vi "settings ui.vi"(10 "ActorConfiguration":T5={"GlobalConfiguration"={"DeviceFamily"="", "WriteData"=FALSE, "BufferSize_samples"=-1, "SyncDevice"=FALSE, "ExecuteInterruptRoutine"=FALSE, "InterruptRoutineTimeout_ms"=-1}, "DeviceConfiguration"={"DeviceSpecificName"="MIPI_Camera", "HardwareReference"="PXIe-Slot2", "UsedResources"=[{"ResourceLocation"="FrontFacing", "ResourceData"=variant(string "Use this Variant to store your specific resource data.\nThis will be read from and written to with the JSON parsing API.\nIn the child implementation you can use the acessors provided to convert from the specific cluster to your own device's implementation")}]}}, 11 "Template":refnum<class "Template.lvclass">) -> (0 "error out":errorcluster, 2 "ActorConfiguration":T5={"GlobalConfiguration"={"DeviceFamily"="", "WriteData"=FALSE, "BufferSize_samples"=-1, "SyncDevice"=FALSE, "ExecuteInterruptRoutine"=FALSE, "InterruptRoutineTimeout_ms"=-1}, "DeviceConfiguration"={"DeviceSpecificName"="MIPI_Camera", "HardwareReference"="PXIe-Slot2", "UsedResources"=[{"ResourceLocation"="FrontFacing", "ResourceData"=variant(string "Use this Variant to store your specific resource data.\nThis will be read from and written to with the JSON parsing API.\nIn the child implementation you can use the acessors provided to convert from the specific cluster to your own device's implementation")}]}})   [LabVIEW 2020, in "Template.lvlib" / "Template.lvclass"]
doc: "Overrides the UI implementation of the settings definition.\nReturns the new configuration for the update settings.vi method"
uses:
  Template.lvclass
  typedefs/actor configuration.ctl
  typedefs/shared actor configuration.ctl
  typedefs/resource config/device configuration cluster.ctl
  typedefs/resource config/single resource cluster.ctl
  f39a1763-17d9-4e4e-a317-0c97e162ffb7.vi
  f86444c9-f386-4375-ae10-303c8fbaebf9.vi
  <vilib>/JDP Science/JSONtext/JSON text to Variant.vi
  <vilib>/JDP Science/JSONtext/Variant to JSON Text.vi
  <vilib>/JDP Science/JSONtext/LVClass Serializer/JSONtext LVClass Serializer.lvclass
panel:
  in  "Sample Resource Data":T1(array[cluster])
  out "Valid JSON?":bool
  in  "JSON Text":string
  in  "DeviceConfiguration":T2={"DeviceSpecificName"="MIPI_Camera", "HardwareReference"="PXIe-Slot2", "UsedResources"=[{"ResourceLocation"="FrontFacing", "ResourceData"=variant(string "Use this Variant to store your specific resource data.\nThis will be read from and written to with the JSON parsing API.\nIn the child implementation you can use the acessors provided to convert from the specific cluster to your own device's implementation")}]}
  in  "GlobalConfiguration":T4={"DeviceFamily"="", "WriteData"=FALSE, "BufferSize_samples"=-1, "SyncDevice"=FALSE, "ExecuteInterruptRoutine"=FALSE, "InterruptRoutineTimeout_ms"=-1}
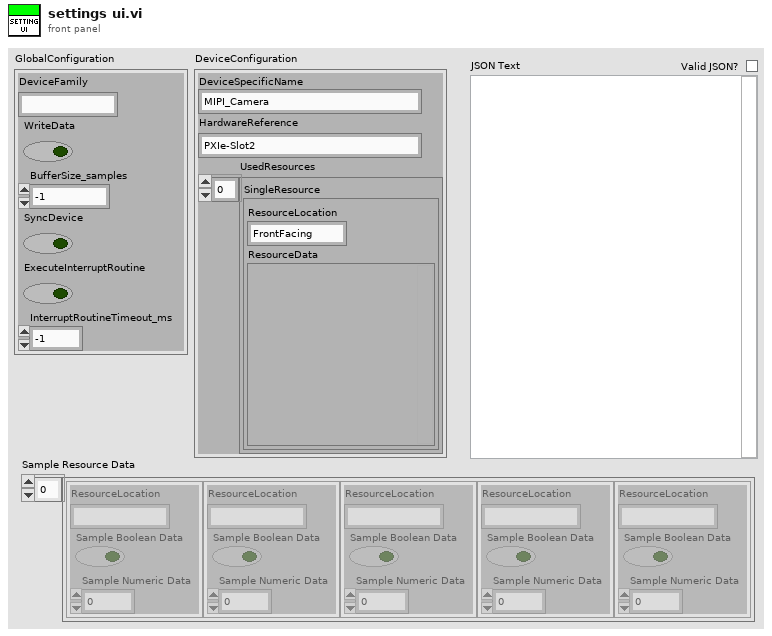
[diagram p1: front panel]
types:
  T1 = cluster{"ResourceLocation":string, "Sample Boolean Data":bool, "Sample Numeric Data":i32}[]
  T2 = typedef "Template.lvlib/Template.lvclass/device configuration cluster.ctl" = cluster{"DeviceSpecificName":string, "HardwareReference":string, "UsedResources":T3[]}
  T3 = typedef "Template.lvlib/Template.lvclass/single resource cluster.ctl" = cluster{"ResourceLocation":string, "ResourceData":variant}
  T4 = typedef "Template.lvlib/Template.lvclass/shared actor configuration.ctl" = cluster{"DeviceFamily":string, "WriteData":bool, "BufferSize_samples":i32, "SyncDevice":bool, "ExecuteInterruptRoutine":bool, "InterruptRoutineTimeout_ms":i32}
  T5 = typedef "Template.lvlib/Template.lvclass/actor configuration.ctl" = cluster{"GlobalConfiguration":T4, "DeviceConfiguration":T2}
  T6 = cluster{"Sample Boolean Data":bool, "Sample Numeric Data":i32}
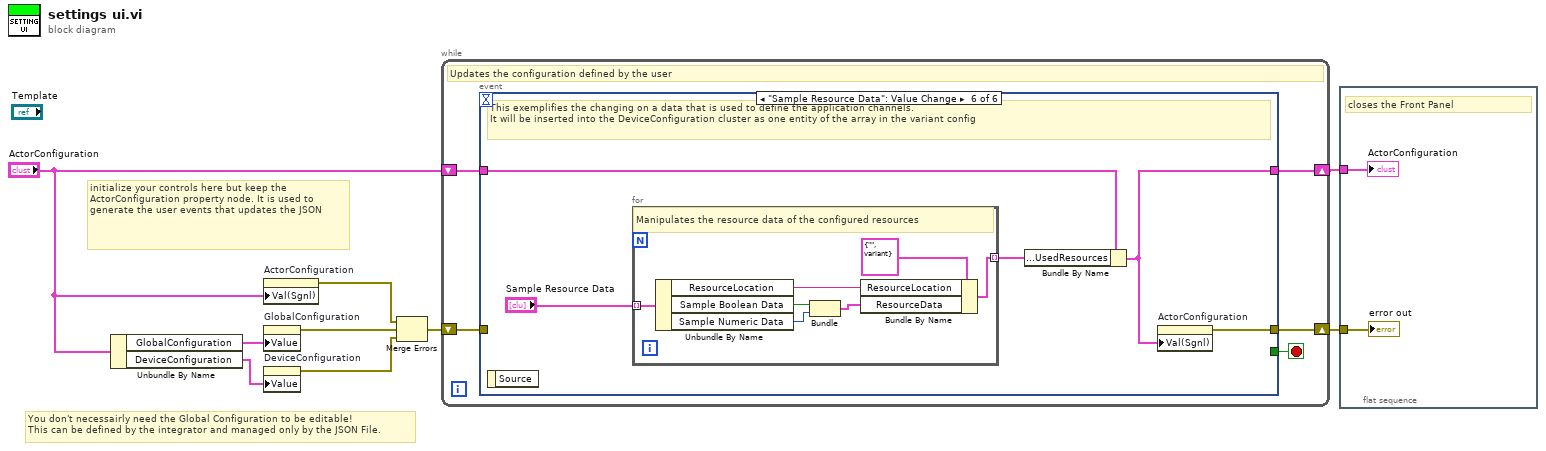
[diagram p0: block diagram]
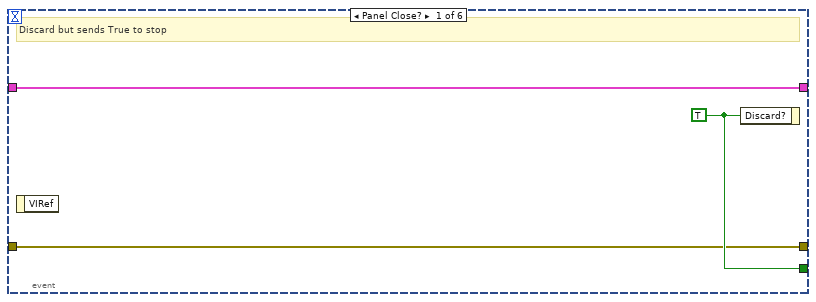
[diagram p2: hidden frame]
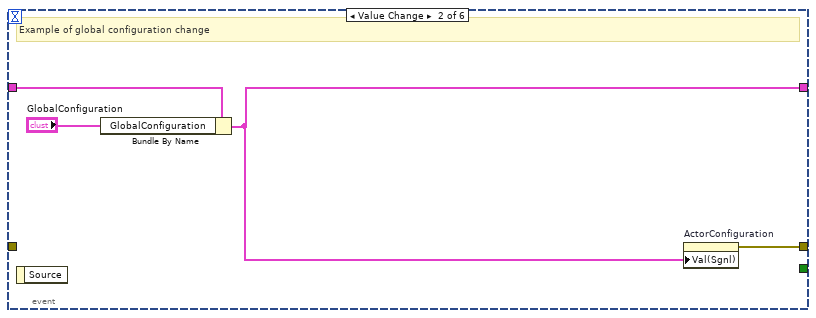
[diagram p3: hidden frame]
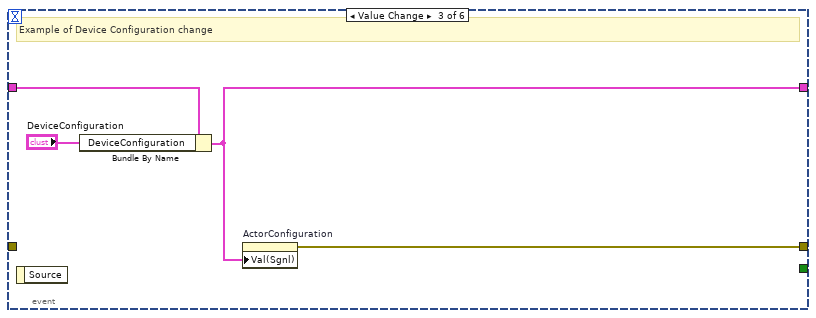
[diagram p4: hidden frame]
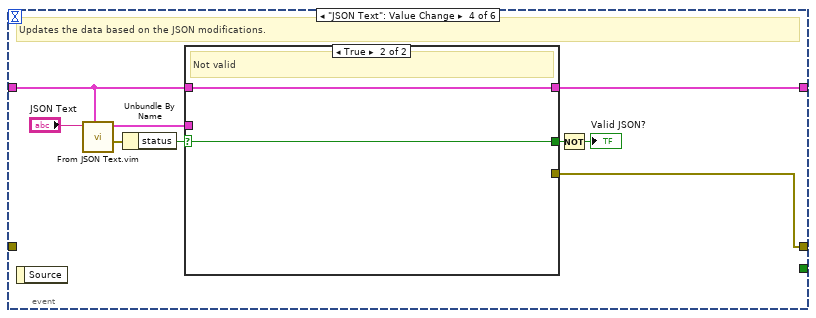
[diagram p5: hidden frame]
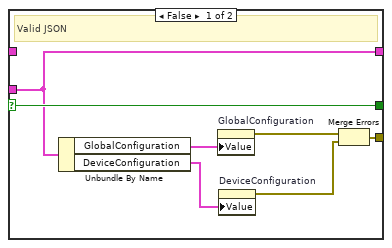
[diagram p6: hidden frame]
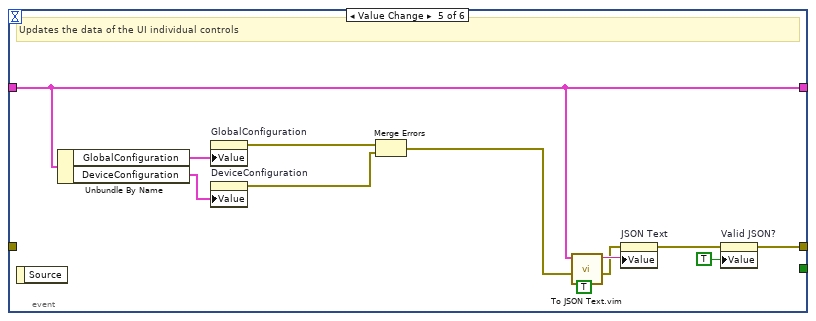
[diagram p7: hidden frame]
diagram:
  # "You don't necessairly need the Global Configuration to be editable!\nThis can be defined by the integrator and managed only by the JSON File."
  # "initialize your controls here but keep the ActorConfiguration property node. It is used to generate the user events that updates the JSON"
  n1 = Unbundle By Name("ActorConfiguration") -> ("GlobalConfiguration"=w7:T4, "DeviceConfiguration"=w5:T2)
  n2 = property on="ActorConfiguration" class="Clust (strict)"("Val(Sgnl)"="ActorConfiguration") -> (error out=w1:errorcluster)  [unwired: 2 in, 1 out]
  n3 = property on="GlobalConfiguration" class="Clust (strict)"("Value"=w7) -> (error out=w6:errorcluster)  [unwired: 2 in, 1 out]
  n4 = property on="DeviceConfiguration" class="Clust (strict)"("Value"=w5) -> (error out=w3:errorcluster)  [unwired: 2 in, 1 out]
  n5 = Merge Errors(w1, w6, w3) -> (w4:errorcluster)
  n6 = while {
    shift-right: [w14] -> w9
    shift-left: "ActorConfiguration" -> [w13]
    shift-right: [w12] -> w8
    shift-left: w4 -> [w10]
    stop <- w11 stop-if-true
    # "Updates the configuration defined by the user"
    n7 = event shown="[5] \"Sample Resource Data\": Value Change" {
      selector: _ -> [_ _ _ _ _ _]
      dyn-events: _ -> [_ _ _ _ _ _]
      timeout: _ -> [_ _ _ _ _ _]
      tunnel: [w17 w18 w22 w32 w47 w58] -> w14
      tunnel: w13 -> [w17 w21 w25 w30 w47 w60]
      tunnel: [w15 w19 w23 w26 w50 w59] -> w12
      tunnel: [w16 _ _ _ _ _] -> w11
      tunnel: w10 -> [w15 _ _ _ _ _]
      event Panel Close? {
        w16 = TRUE ("Discard?")
        # "Discard but sends True to stop"
        n8 = event-data() -> ()  [unwired: 1 in, 1 out]
        n9 = event-data("Discard?"=w16) -> ()  [unwired: 1 in, 1 out]
      }
      event Value Change {
        # "Example of global configuration change"
        n10 = event-data() -> ()  [unwired: 1 in, 1 out]
        n11 = Bundle By Name(cluster=w21, "GlobalConfiguration"="GlobalConfiguration") -> (w18:T5)
        n12 = property on="ActorConfiguration" class="Clust (strict)"("Val(Sgnl)"=w18) -> (error out=w19:errorcluster)  [unwired: 2 in, 1 out]
      }
      event Value Change {
        # "Example of Device Configuration change"
        n13 = event-data() -> ()  [unwired: 1 in, 1 out]
        n14 = Bundle By Name(cluster=w25, "DeviceConfiguration"="DeviceConfiguration") -> (w22:T5)
        n15 = property on="ActorConfiguration" class="Clust (strict)"("Val(Sgnl)"=w22) -> (error out=w23:errorcluster)  [unwired: 2 in, 1 out]
      }
      event "JSON Text": Value Change {
        # "Updates the data based on the JSON modifications."
        n16 = event-data() -> ()  [unwired: 1 in, 1 out]
        n17 = call "From JSON Text.vim"("Data Type and Default Value"=w30, "JSON"="JSON Text") -> ("error out"=w33:errorcluster, "Data out"=w31:T5)  [unwired: 8 in]
        n18 = Unbundle By Name(w33) -> ("status"=w29:bool)
        n19 = case shown="True" w29 {
          selector: w29 -> [w41 w42]
          tunnel: [w40 w43] -> w32
          tunnel: w31 -> [w40 _]
          tunnel: w30 -> [_ w43]
          tunnel: [w41 w42] -> w28
          tunnel: [w35 _] -> w26
          frame False {
            # "Valid JSON"
            n20 = Unbundle By Name(w40) -> ("GlobalConfiguration"=w39:T4, "DeviceConfiguration"=w38:T2)
            n21 = property on="GlobalConfiguration" class="Clust (strict)"("Value"=w39) -> (error out=w37:errorcluster)  [unwired: 2 in, 1 out]
            n22 = property on="DeviceConfiguration" class="Clust (strict)"("Value"=w38) -> (error out=w36:errorcluster)  [unwired: 2 in, 1 out]
            n23 = Merge Errors(w37, w36) -> (w35:errorcluster)
          }
          frame True {
            # "Not valid"
          }
        }
        n24 = Not(x=w28) -> (.not. x?=→"Valid JSON?":bool)
      }
      event Value Change {
        # "Updates the data of the UI individual controls"
        n25 = event-data() -> ()  [unwired: 1 in, 1 out]
        n26 = Unbundle By Name(w47) -> ("GlobalConfiguration"=w48:T4, "DeviceConfiguration"=w49:T2)
        n27 = property on="GlobalConfiguration" class="Clust (strict)"("Value"=w48) -> (error out=w46:errorcluster)  [unwired: 2 in, 1 out]
        n28 = property on="DeviceConfiguration" class="Clust (strict)"("Value"=w49) -> (error out=w44:errorcluster)  [unwired: 2 in, 1 out]
        n29 = Merge Errors(w46, w44) -> (w45:errorcluster)
        n30 = call "To JSON Text.vim"("Pretty Print?"=TRUE, "error in (no error)"=w45, "Anything"=w47) -> ("error out"=w53:errorcluster, "<JSON>"=w54:string)  [unwired: 7 in]
        n31 = property on="JSON Text" class="Str"(error in=w53, "Value"=w54) -> (error out=w51:errorcluster)  [unwired: 1 in, 1 out]
        n32 = property on="Valid JSON?" class="Bool (strict)"(error in=w51, "Value"=TRUE ("Valid JSON?")) -> (error out=w50:errorcluster)  [unwired: 1 in, 1 out]
      }
      event "Sample Resource Data": Value Change {
        # "This exemplifies the changing on a data that is used to define the application channels.\nIt will be inserted into the DeviceConfiguration cluster as one entity of the array in the variant config"
        n33 = event-data() -> ()  [unwired: 1 in, 1 out]
        n34 = for {
          tunnel: "Sample Resource Data" -> [w67] mode=indexing
          tunnel: [w66] -> w56 mode=indexing
          # "Manipulates the resource data of the configured resources"
          n35 = Unbundle By Name(w67) -> ("ResourceLocation"=w65:string, "Sample Boolean Data"=w64:bool, "Sample Numeric Data"=w63:i32)
          n36 = Bundle("Sample Boolean Data"=w64, "Sample Numeric Data"=w63) -> (w62:T6)  [unwired: 1 in]
          n37 = Bundle By Name(cluster=T3 {"ResourceLocation"="", "ResourceData"=variant} ("SingleResource"), "ResourceLocation"=w65, "ResourceData"=w62) -> (w66:T3)
        }
        n38 = Bundle By Name(cluster=w60, "DeviceConfiguration.UsedResources"=w56) -> (w58:T5)
        n39 = property on="ActorConfiguration" class="Clust (strict)"("Val(Sgnl)"=w58) -> (error out=w59:errorcluster)  [unwired: 2 in, 1 out]
      }
    }
  }
  n40 = flat-sequence {
    tunnel: w9 -> [w69]
    tunnel: w8 -> [w68]
    frame #0 {
      # "closes the Front Panel"
      "error out" <- w68
      "ActorConfiguration" <- w69
    }
  }
